vi "Handle Persistent Fields.vi"(9 "Field IDs":T1[](array[typedef]), 10 "Field ID":T1, 11 "Operation":T2(ring)) -> (1 "Field IDs out":T1[](array[typedef]))   [LabVIEW 2017]
uses:
  <vilib>/Rock Robotics/Network Tables/Field ID.ctl
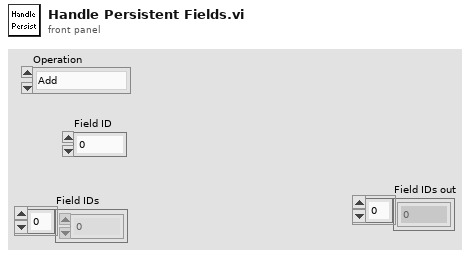
[diagram p1: front panel]
types:
  T1 = typedef "Field ID.ctl" = i32
  T2 = enum16{"Add", "Remove", "Clear", "Init", "Retrieve"}
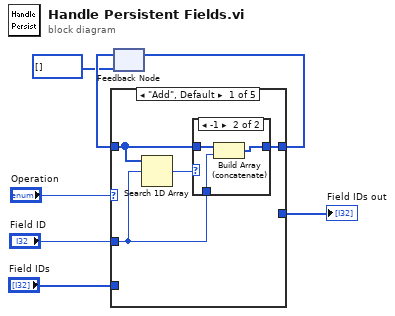
[diagram p0: block diagram]
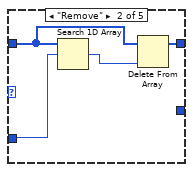
[diagram p3: hidden frame]
diagram:
  n1 = feedback #1(T1[] [] ("Field IDs")) -> (w6:T1[])
  n2 = case shown="\"Add\", Default" "Operation" {
    tunnel: w6 -> [w10 w18 _ _ w21]
    tunnel: [w11 w16 _ w20 w21] -> w5
    tunnel: "Field IDs" -> [_ _ _ w20 _]
    tunnel: "Field ID" -> [w9 w19 _ _ _]
    tunnel: [_ _ _ _ w21] -> w1
    frame "Add", Default {
      n3 = Search 1D Array(1D array=w10, element=w9) -> (index of element=w8:i32)  [unwired: 1 in]
      n4 = case shown="-1" w8 {
        tunnel: [w12 w15] -> w11
        tunnel: w10 -> [w12 w14]
        tunnel: w9 -> [_ w13]
        frame Default {
        }
        frame -1 {
          n5 = Build Array (concatenate)(w14, w13) -> (w15:T1[])
        }
      }
    }
    frame "Remove" {
      n6 = Search 1D Array(1D array=w18, element=w19) -> (index of element=w17:i32)  [unwired: 1 in]
      n7 = Delete From Array(array=w18, index=w17) -> (array with subset deleted=w16:T1[])  [unwired: 1 in, 1 out]
    }
    frame "Clear" {
    }
    frame "Init" {
    }
    frame "Retrieve" {
    }
  }
  "Field IDs out" <- w1
  n8 = feedback-in #1(w5) -> ()
